vi "Cut overscan area from file.vi"() -> ()   [LabVIEW 2021]
doc: "This VI allows loading an sxm file, removing a user-defined overscan area from the data, and saving a new sxm file with the new calculated data."
uses:
  Nanonis Prog Interface.lvlib
panel:
  in  "Total Overscan":cluster{"% pixels":u32, "% lines":u32}={"% pixels"=10, "% lines"=10}
  in  "Scan Data File Path":path
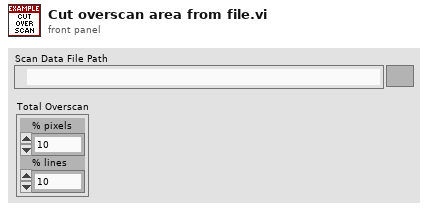
[diagram p1: front panel]
types:
  T1 = cluster{"Number of channels":i8, "Config":cluster{"Name":string, "Calibration":sgl, "Offset":sgl}[]}
  T2 = cluster{"center X":sgl, "center Y":sgl, "angle":sgl, "width":sgl, "height":sgl, "# pixels":i32, "# lines":i32}
  T3 = cluster{"up/down":bool, "time/line":sgl, "starttime":timestamp, "endtime":timestamp}
  T4 = cluster{"Name":string, "Calibration":sgl, "Offset":sgl}[]
  T5 = cluster{"Name":string, "Calibration":sgl, "Offset":sgl, "Channel index":i32}
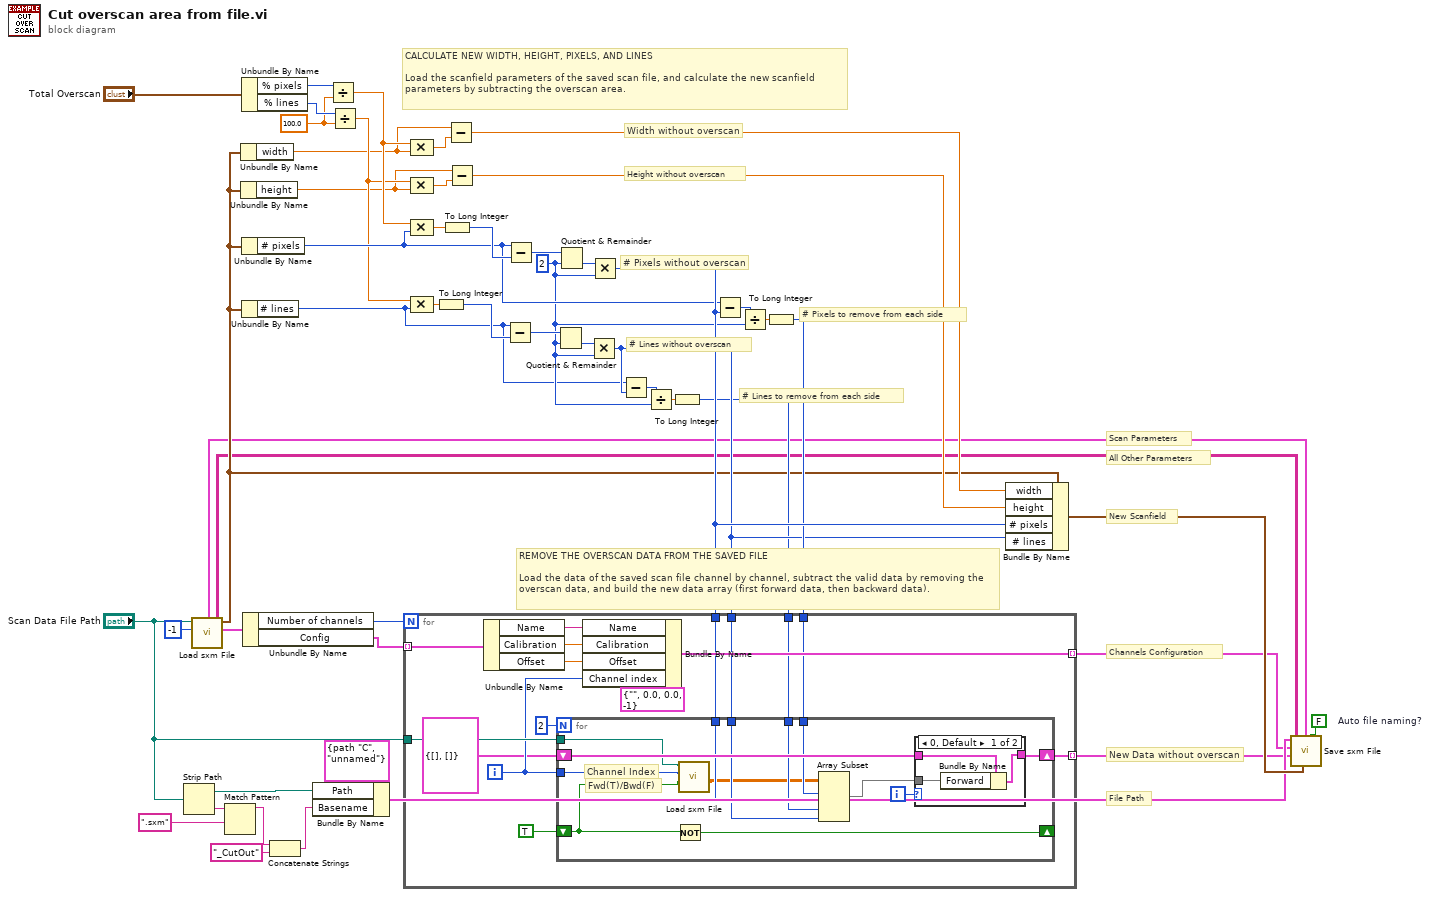
[diagram p0: block diagram]
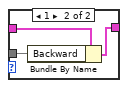
[diagram p2: hidden frame]
diagram:
  w21 = 2 ("y")
  w22 = sgl 100.0 ("y")
  w7 = FALSE  # Auto file naming?
  # "File Path"
  # "All Other Parameters"
  # "Scan Parameters"
  # "New Data without overscan"
  # "Channels Configuration"
  # "New Scanfield"
  # "# Pixels without overscan"
  # "# Pixels to remove from each side"
  # "# Lines without overscan"
  # "# Lines to remove from each side"
  # "Width without overscan"
  # "Height without overscan"
  # "REMOVE THE OVERSCAN DATA FROM THE SAVED FILE\n\nLoad the data of the saved scan file channel by channel, subtract the valid data by removing the overscan data, and build the new data array (first forward data, then backward data)."
  # "CALCULATE NEW WIDTH, HEIGHT, PIXELS, AND LINES\n\nLoad the scanfield parameters of the saved scan file, and calculate the new scanfield parameters by subtracting the overscan area."
  n1 = Strip Path(path="Scan Data File Path") -> (stripped path=w48:path, name=w47:string)
  n2 = call "Load sxm File.vi"("Read channel"=i8 -1, "Scan data file"="Scan Data File Path") -> ("Channels info"=w8:T1, "Scanfield"=w9:T2, "Parameters"=w1:string[][], "Scan param"=w2:T3)  [unwired: 4 in, 2 out]
  n3 = Match Pattern(string=w47, regular expression=".sxm") -> (before substring=w45:string)  [unwired: 1 in, 3 out]
  n4 = Unbundle By Name(w9) -> ("width"=w17:sgl)
  n5 = Unbundle By Name(w9) -> ("height"=w15:sgl)
  n6 = Unbundle By Name("Total Overscan") -> ("% pixels"=w26:u32, "% lines"=w25:u32)
  n7 = Unbundle By Name(w9) -> ("# pixels"=w27:i32)
  n8 = Unbundle By Name(w9) -> ("# lines"=w18:i32)
  n9 = Unbundle By Name(w8) -> ("Number of channels"=w51:i8, "Config"=w50:T4)
  n10 = Concatenate Strings(w45, "_CutOut" ("string")) -> (w44:string)
  n11 = Bundle By Name(cluster=cluster{"Path":path, "Basename":string} {"Path"=path "C:/", "Basename"="unnamed"} ("Filename control"), "Path"=w48, "Basename"=w44) -> (w5:cluster{"Path":path, "Basename":string})
  n12 = Divide(x=w26, y=w22) -> (x/y=w20:sgl)
  n13 = Divide(x=w25, y=w22) -> (x/y=w19:sgl)
  n14 = Compound Arithmetic op=MULTIPLY(w20, w17) -> (w16:sgl)
  n15 = Compound Arithmetic op=MULTIPLY(w19, w15) -> (w14:sgl)
  n16 = Compound Arithmetic op=MULTIPLY(w20, w27) -> (w41:sgl)
  n17 = Compound Arithmetic op=MULTIPLY(w19, w18) -> (w28:sgl)
  n18 = To Long Integer(number=w28) -> (32bit integer=w29:i32)
  n19 = To Long Integer(number=w41) -> (32bit integer=w40:i32)
  n20 = Subtract(x=w17, y=w16) -> (x-y=w13:sgl)
  n21 = Subtract(x=w15, y=w14) -> (x-y=w12:sgl)
  n22 = Subtract(x=w18, y=w29) -> (x-y=w30:i32)
  n23 = Subtract(x=w27, y=w40) -> (x-y=w39:i32)
  n24 = Quotient & Remainder(x=w30, y=w21) -> (floor(x/y)=w31:i32)  [unwired: 1 out]
  n25 = Quotient & Remainder(x=w39, y=w21) -> (floor(x/y)=w38:i32)  [unwired: 1 out]
  n26 = Multiply(x=w31, y=w21) -> (x*y=w24:i32)
  n27 = Multiply(x=w38, y=w21) -> (x*y=w35:i32)
  n28 = Subtract(x=w18, y=w24) -> (x-y=w32:i32)
  n29 = Divide(x=w32, y=w21) -> (x/y=w33:dbl)
  n30 = To Long Integer(number=w33) -> (32bit integer=w23:i32)
  n31 = Subtract(x=w27, y=w35) -> (x-y=w37:i32)
  n32 = Divide(x=w37, y=w21) -> (x/y=w36:dbl)
  n33 = To Long Integer(number=w36) -> (32bit integer=w34:i32)
  n34 = for {
    N: w51 -> [_]
    tunnel: "Scan Data File Path" -> [w67]
    tunnel: [w64] -> w3 mode=indexing
    tunnel: w50 -> [w63] mode=indexing
    tunnel: [w58] -> w4 mode=indexing
    tunnel: w35 -> [w55]
    tunnel: w34 -> [w54]
    tunnel: w24 -> [w53]
    tunnel: w23 -> [w52]
    i -> [w59]
    n35 = Unbundle By Name(w63) -> ("Name"=w62:string, "Calibration"=w61:sgl, "Offset"=w60:sgl)
    n36 = for {
      N: 2 -> [_]
      tunnel: w67 -> [w71]
      tunnel: w59 -> [w70]
      shift-right: [w80] -> _
      shift-left: TRUE -> [w69]
      shift-right: [w78] -> w64
      shift-left: cluster{"Forward":sgl[][], "Backward":sgl[][]} {"Forward"=[], "Backward"=[]} -> [w77]
      tunnel: w55 -> [w75]
      tunnel: w54 -> [w74]
      tunnel: w53 -> [w73]
      tunnel: w52 -> [w72]
      i -> [w79]
      # "Channel Index"
      # "Fwd(T)/Bwd(F)"
      n37 = Not(x=w69) -> (.not. x?=w80:bool)
      n38 = call "Load sxm File.vi"("Scan direction"=w69, "Read channel"=w70, "Scan data file"=w71) -> ("Data"=w68:sgl[][])  [unwired: 3 in, 5 out]
      n39 = Array Subset(array=w68, index (row)=w74, length (row)=w75, index (col)=w72, length (col)=w73) -> (w76:sgl[][])
      n40 = case shown="0, Default" w79 {
        tunnel: w76 -> [w83 w86]
        tunnel: [w82 w85] -> w78
        tunnel: w77 -> [w81 w84]
        frame 0, Default {
          n41 = Bundle By Name(cluster=w81, "Forward"=w83) -> (w82:cluster{"Forward":sgl[][], "Backward":sgl[][]})
        }
        frame 1 {
          n42 = Bundle By Name(cluster=w84, "Backward"=w86) -> (w85:cluster{"Forward":sgl[][], "Backward":sgl[][]})
        }
      }
    }
    n43 = Bundle By Name(cluster=T5 {"Name"="", "Calibration"=0.0, "Offset"=0.0, "Channel index"=-1} ("channel config"), "Name"=w62, "Calibration"=w61, "Offset"=w60, "Channel index"=w59) -> (w58:T5)
  }
  n44 = Bundle By Name(cluster=w9, "width"=w13, "height"=w12, "# pixels"=w35, "# lines"=w24) -> (w6:T2)
  n45 = call "Save sxm File.vi"("Parameters"=w1, "Auto file naming? (T)"=w7, "Scanfield"=w6, "Scan param"=w2, "Channels data"=w3, "Channels config"=w4, "Filename control"=w5) -> ()  [unwired: 2 in, 3 out]
